vi "Stop Core.vi"(10 "final error code":i32, 11 "CS++DeviceGUIActor in":refnum<class "CS++GUIActor.lvclass">) -> (3 "CS++DeviceGUIActor out":refnum<class "CS++GUIActor.lvclass">)   [LabVIEW 2012, in "CS++GUIActor.lvlib" / "CS++GUIActor.lvclass"]
doc: "(<B>Filename</B>: Actor Framework.lvlib:Actor.lvclass:Stop Core.vi)\n\nDefines what the actor does before it stops. Use the <B>final error code</B> input to determine whether the actor shut down in response to an error.\n\nBy default, this method does nothing. A descendant class may override it to define behavior, such as shutting down any processes the actor initiated in its override of the Actor Core method."
uses:
  CS++GUIActor.lvclass
  CS++BaseActor/CS++BaseActor.lvclass
  CS++GUIActor.lvclass/CS++GUIActor.ctl
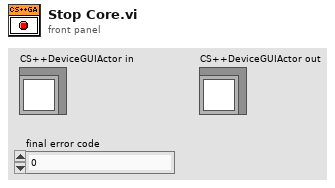
[diagram p1: front panel]
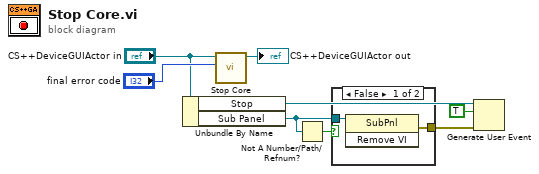
[diagram p0: block diagram]
diagram:
  n1 = Unbundle By Name("CS++DeviceGUIActor in") -> ("Stop"=w5:refnum<user-event>, "Sub Panel"=w1:refnum<vi>)
  n2 = call-parent "Stop Core.vi"("final error code"="final error code", "CS++BaseActor in"="CS++DeviceGUIActor in") -> ("CS++BaseActor out"=→"CS++DeviceGUIActor out":refnum<class "CS++GUIActor.lvclass">)  [unwired: 9 in]
  n3 = Not A Number/Path/Refnum?(number/path/refnum=w1) -> (NaN/Path/Refnum?=w2:bool)
  n4 = case shown="False" w2 {
    tunnel: w1 -> [w10 _]
    tunnel: [w9 _] -> w3
    frame False {
      n5 = invoke class="SubPnl" method="Remove VI"(reference=w10) -> (error out=w9:errorcluster)  [unwired: 2 in, 2 out]
    }
    frame True {
    }
  }
  n6 = Generate User Event(user event=w5, event data cluster=TRUE ("event data"), error in=w3) -> ()  [unwired: 2 out]
